vi "IniToken Write To LabVIEW.ini.vi"(8 "error in (no error)":errorcluster, 11 "Cluster":cluster{"IniTokenCluster":T1, "Items":string[]}) -> (0 "error out":errorcluster)   [LabVIEW 2012]
uses:
  Def-IniTokenCluster.ctl
  <resource>/dialog/lvconfig.llb/LV Config Read String.vi
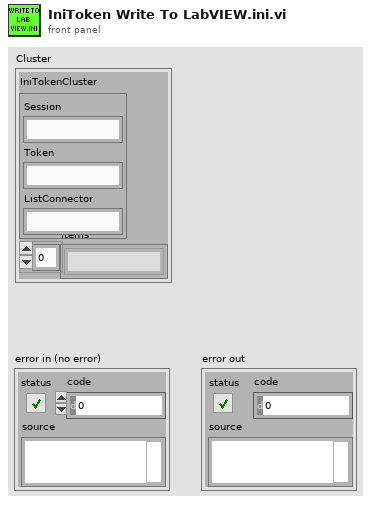
[diagram p1: front panel]
types:
  T1 = typedef "Def-IniTokenCluster.ctl" = cluster{"Session":string, "Token":string, "ListConnector":string}
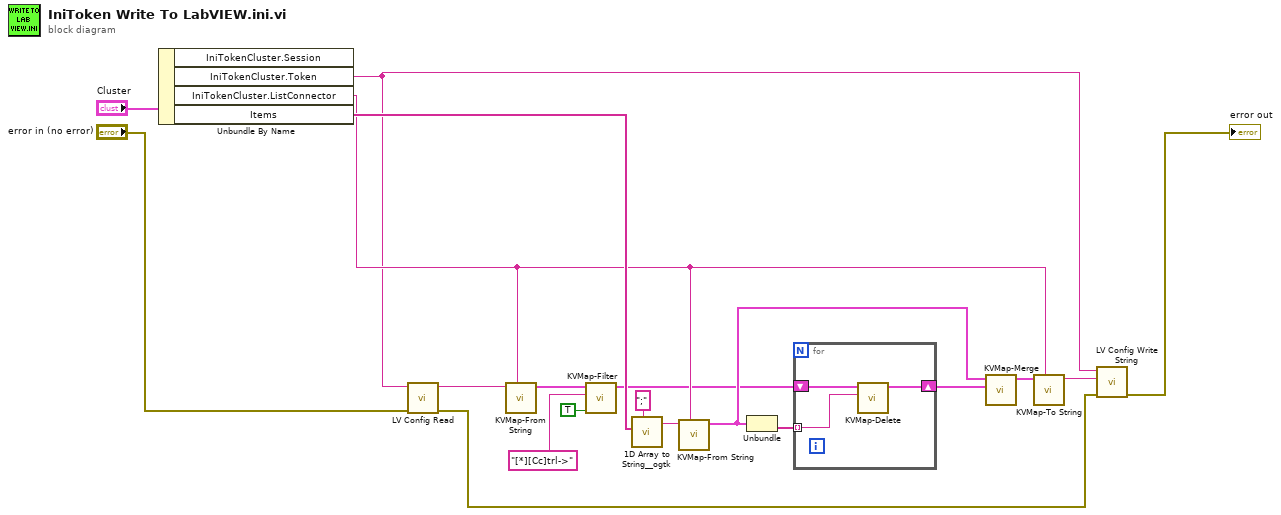
[diagram p0: block diagram]
diagram:
  n1 = Unbundle By Name("Cluster") -> ("IniTokenCluster.Token"=w1:string, "IniTokenCluster.ListConnector"=w13:string, "Items"=w14:string[])  [unwired: 1 out]
  n2 = call-poly <resource>:"LV Config Read.vi"("error in"="error in (no error)", "key"=w1) -> ("error out"=w18:errorcluster, "value"=w2:string)  [unwired: 3 in, 1 out]
  n3 = call "KVMap-From String.vi"("delimiter (Tab)"=w13, "value"=w2) -> ("Cluster"=w3:cluster{string[], string[]})  [unwired: 9 in]
  n4 = call "KVMap-Filter.vi"("T->First/F->Second(F)"=TRUE, "filter"="[*][Cc]trl->", "Cluster in"=w3) -> ("Cluster out"=w6:cluster{string[], string[]})  [unwired: 8 in]
  n5 = call <userlib>:"1D Array to String__ogtk.vi"("delimiter (Tab)"=";", "Array of Strings"=w14) -> ("delimited string"=w16:string)  [unwired: 9 in]
  n6 = call "KVMap-From String.vi"("delimiter (Tab)"=w13, "value"=w16) -> ("Cluster"=w9:cluster{string[], string[]})  [unwired: 9 in]
  n7 = Unbundle(w9) -> (w7:string[])  [unwired: 1 out]
  n8 = for {
    shift-right: [w21] -> w8
    shift-left: w6 -> [w22]
    tunnel: w7 -> [w20] mode=indexing
    n9 = call "KVMap-Delete.vi"("element"=w20, "Cluster in"=w22) -> ("Cluster out"=w21:cluster{string[], string[]})  [unwired: 9 in]
  }
  n10 = call "KVMap-Merge.vi"("Cluster 2"=w8, "Cluster in"=w9) -> ("Cluster"=w10:cluster{string[], string[]})  [unwired: 8 in]
  n11 = call "KVMap-To String.vi"("string"=w13, "Cluster"=w10) -> ("value"=w11:string)  [unwired: 9 in]
  n12 = call <resource>:"LV Config Write String.vi"("error in (no error)"=w18, "value"=w11, "key"=w1) -> ("error out"=→"error out":errorcluster)  [unwired: 4 in]
